vi "rotatePoints.vi"(7 "robotPos":cluster{"xPos":dbl, "yPos":dbl, "theta":dbl}, 9 "angle shift":dbl, 10 "Input":cluster{"Line":cluster{"X":dbl, "Y":dbl}[]}[](array[cluster])=[{"Line"=[{"X"=2207.719904848649, "Y"=4025.6413471932437}, {"X"=2198.7079256765874, "Y"=4062.926864756568}, {"X"=2207.699360265736, "Y"=4067.8159613100943}, {"X"=2234.0955267399086, "Y"=4039.9831033175988}, {"X"=2252.228831694671, "Y"=4026.9405312945887}, {"X"=2271.549062590683, "Y"=4011.064573925477}, {"X"=2281.5806891164716, "Y"=4012.833569019945}, {"X"=2291.606547380772, "Y"=4014.532684771267}, {"X"=2306.491333736606, "Y"=4006.2964587232555}, {"X"=2318.6274797470815, "Y"=4003.328717244889}, {"X"=2330.269715175642, "Y"=4001.167493766924}, {"X"=2341.008251095636, "Y"=4000.7261955414297}, {"X"=2355.4973825011707, "Y"=3992.0389276299557}, {"X"=2366.5383203403635, "Y"=3990.5072097629672}, {"X"=2377.53610248222, "Y"=3988.892615102757}, {"X"=2388.8934994574606, "Y"=3986.2805794624155}, {"X"=2397.411061091578, "Y"=3990.0041621179494}, {"X"=2407.911866591801, "Y"=3989.075823084253}, {"X"=2418.3785187827534, "Y"=3988.071126631001}, {"X"=2427.2873049759087, "Y"=3990.6890985976133}, {"X"=2437.3316429744427, "Y"=3990.4691007002493}, {"X"=2446.612827733287, "Y"=3992.036866455286}, {"X"=2458.074290966777, "Y"=3987.9540791715117}, {"X"=2466.9588047209436, "Y"=3990.3194180243167}, {"X"=2475.8519286932046, "Y"=3992.628019014901}, {"X"=2486.4858053530056, "Y"=3990.1896172450897}, {"X"=2497.4106848755673, "Y"=3986.733204449491}, {"X"=2506.263944361786, "Y"=3988.8486985135632}, {"X"=2516.111756914983, "Y"=3988.0749865205753}, {"X"=2525.2846850863148, "Y"=3989.1253974304846}, {"X"=2533.8171346698073, "Y"=3992.0120459509435}, {"X"=2542.367135774692, "Y"=3994.846286004641}, {"X"=2550.9343664982594, "Y"=3997.6280108840406}, {"X"=2559.8185598039045, "Y"=3999.4031941177254}, {"X"=2571.9437832226267, "Y"=3990.6088146125935}, {"X"=2582.2144175424637, "Y"=3987.463948032747}, {"X"=2590.735600977976, "Y"=3990.0013135580634}, {"X"=2599.5487477190327, "Y"=3991.5253481509435}, {"X"=2609.718442836895, "Y"=3988.1802138549383}, {"X"=2620.6261722825793, "Y"=3981.8699283373353}, {"X"=2630.4064035936003, "Y"=3979.3420799407895}, {"X"=2639.129732346304, "Y"=3980.6164021637396}, {"X"=2647.6078286155175, "Y"=3982.8046707857657}, {"X"=2656.099192250811, "Y"=3984.9408775935008}, {"X"=2664.6035035571426, "Y"=3987.0249421599656}, {"X"=2673.807645346353, "Y"=3986.136554516008}, {"X"=2686.7807721936474, "Y"=3968.6159853415393}]}, {"Line"=[{"X"=3111.693546822526, "Y"=3588.7110556670254}, {"X"=3123.438852104627, "Y"=3635.669759040541}, {"X"=3147.3373670544443, "Y"=3774.796876174543}, {"X"=3159.6335330851234, "Y"=3812.53706546017}, {"X"=3170.3490866292254, "Y"=3835.3097541445177}, {"X"=3179.3524271873403, "Y"=3844.1389419441903}, {"X"=3195.610637480107, "Y"=3900.369746843038}, {"X"=3206.0629644143296, "Y"=3914.952111180015}, {"X"=3215.736251259236, "Y"=3923.5327233931966}, {"X"=3223.853234205395, "Y"=3922.1840755113426}, {"X"=3233.691556461108, "Y"=3930.6349072674984}, {"X"=3245.0740830877103, "Y"=3946.885182114169}, {"X"=3253.3338017504625, "Y"=3945.356081076923}, {"X"=3263.30367270885, "Y"=3952.6105041504115}, {"X"=3271.5981781203227, "Y"=3950.96944067648}, {"X"=3279.8824580138976, "Y"=3949.2775139666783}, {"X"=3287.319752884467, "Y"=3943.6232208481697}, {"X"=3295.558661266366, "Y"=3941.8349666596237}, {"X"=3303.7864420317183, "Y"=3939.9961931429916}, {"X"=3311.3215566201256, "Y"=3935.1853385892246}, {"X"=3319.508239302628, "Y"=3933.249970942334}, {"X"=3334.3751764114004, "Y"=3958.45288523373}]}, {"Line"=[{"X"=3344.908865242611, "Y"=3965.101415528185}, {"X"=3352.2748452131286, "Y"=3959.0873531271145}, {"X"=3360.607416965633, "Y"=3956.9002508767453}, {"X"=3369.977484451716, "Y"=3958.521498173209}, {"X"=3378.3062509363144, "Y"=3956.2257852225457}, {"X"=3389.641249204419, "Y"=3964.456190912123}, {"X"=3400.249927965521, "Y"=3969.718582469989}, {"X"=3408.646828597577, "Y"=3967.236910515929}, {"X"=3417.0283439075047, "Y"=3964.703762864954}, {"X"=3425.39415833599, "Y"=3962.11923488864}, {"X"=3433.7439569148473, "Y"=3959.483423893006}, {"X"=3442.07742527888, "Y"=3956.7964291148455}, {"X"=3453.8661044404716, "Y"=3964.496082530115}, {"X"=3462.5513905712496, "Y"=3962.632456343457}, {"X"=3471.2308824116985, "Y"=3960.7135831840187}, {"X"=3479.5711932104623, "Y"=3957.796549797757}, {"X"=3489.5875228985537, "Y"=3959.5326614031965}, {"X"=3499.987731033616, "Y"=3962.1355544936987}, {"X"=3509.7375659322042, "Y"=3962.7885433468805}, {"X"=3522.362789825989, "Y"=3970.848684503585}, {"X"=3531.8497335130646, "Y"=3970.4144850964185}, {"X"=3540.6159427308094, "Y"=3968.055336039182}, {"X"=3549.37321102068, "Y"=3965.6401704009836}, {"X"=3558.500081793643, "Y"=3964.0944463769706}, {"X"=3569.16692785225, "Y"=3966.180444977614}, {"X"=3577.538939065994, "Y"=3962.6623844014066}, {"X"=3585.8892062651075, "Y"=3959.093020356606}, {"X"=3593.8159168133284, "Y"=3954.5566274390844}, {"X"=3602.1161416132213, "Y"=3950.8875423249738}, {"X"=3609.568283021091, "Y"=3945.3458694085766}, {"X"=3618.6482715704797, "Y"=3943.396931693257}, {"X"=3626.8795543024958, "Y"=3939.5756881929083}]}, {"Line"=[{"X"=3800.09423982062, "Y"=3947.3448732250645}, {"X"=3809.378042970595, "Y"=3944.123574511321}, {"X"=3819.694604811834, "Y"=3942.5459972911062}, {"X"=3832.6538504761256, "Y"=3945.14369689163}, {"X"=3843.5495084753843, "Y"=3944.244481763246}, {"X"=3859.2959007671043, "Y"=3950.8558601586074}, {"X"=3868.110312080752, "Y"=3946.3983385532897}, {"X"=3881.8256977872484, "Y"=3949.417444203991}, {"X"=3890.088967448885, "Y"=3943.9812610396684}, {"X"=3903.3341528929327, "Y"=3945.9674617973524}, {"X"=3914.3876190160663, "Y"=3944.533853121642}, {"X"=3929.996733704319, "Y"=3949.602561978636}, {"X"=3938.2602324211293, "Y"=3943.870803409706}, {"X"=3956.3055525432223, "Y"=3951.9673406465863}, {"X"=3970.4078429817587, "Y"=3954.2025765296307}, {"X"=3979.8737146602944, "Y"=3949.841288195704}, {"X"=3998.208687435405, "Y"=3957.499324614376}, {"X"=4008.3113782978594, "Y"=3953.754839103104}, {"X"=4017.8033817005166, "Y"=3949.1390870473633}, {"X"=4027.276658663517, "Y"=3944.457759308607}, {"X"=4044.6867826496114, "Y"=3949.9920467014626}, {"X"=4054.1841976192836, "Y"=3945.1307287731506}, {"X"=4072.364489063383, "Y"=3951.169642419422}, {"X"=4082.5142882560313, "Y"=3946.9026749255263}, {"X"=4105.907771200753, "Y"=3958.849513963111}, {"X"=4114.860669673112, "Y"=3952.809922796259}, {"X"=4127.6252414941555, "Y"=3951.3183617287414}, {"X"=4137.831733452446, "Y"=3946.665491630569}, {"X"=4155.174277321527, "Y"=3950.2967781249745}, {"X"=4169.984998772591, "Y"=3950.7420562961306}, {"X"=4185.503775549924, "Y"=3951.807973847201}, {"X"=4205.727035469534, "Y"=3957.9684517461556}, {"X"=4217.379287768711, "Y"=3954.26314640536}, {"X"=4225.665973398596, "Y"=3946.7679539003266}, {"X"=4237.972103227306, "Y"=3943.6346496093947}, {"X"=4272.112912884239, "Y"=3963.801208707917}, {"X"=4281.830236954413, "Y"=3957.4241207630703}, {"X"=4299.118370011982, "Y"=3958.9302633679963}, {"X"=4309.518481723098, "Y"=3953.0891862791714}, {"X"=4319.8957456070275, "Y"=3947.171563212521}, {"X"=4354.192697994926, "Y"=3965.3172293270245}, {"X"=4369.630150249946, "Y"=3964.0389479506475}, {"X"=4388.666973836772, "Y"=3966.128850356006}, {"X"=4404.194818830778, "Y"=3964.551541997882}, {"X"=4414.705377278174, "Y"=3957.9873694185153}, {"X"=4444.055220504324, "Y"=3969.2350127477052}, {"X"=4461.187873541066, "Y"=3968.5517886497883}, {"X"=4486.44067286851, "Y"=3975.179670458451}, {"X"=4494.850634872708, "Y"=3966.033154583249}, {"X"=4506.915932191928, "Y"=3960.185418722805}, {"X"=4515.233505756106, "Y"=3950.9135512807848}, {"X"=4497.977382829493, "Y"=3919.1208286322008}, {"X"=4462.280379962087, "Y"=3871.8412205845257}, {"X"=4470.0567239687225, "Y"=3862.8448947968027}, {"X"=4477.77772117058, "Y"=3853.8010236125533}, {"X"=4655.602195404125, "Y"=3987.2928207747054}, {"X"=4908.623903346539, "Y"=3991.4736057770633}, {"X"=4938.228890195194, "Y"=3994.923929543366}, {"X"=4946.751495910105, "Y"=3983.004921600703}, {"X"=4955.200807531504, "Y"=3971.0338443044193}, {"X"=4963.576506947583, "Y"=3959.011148358809}, {"X"=4995.824874331277, "Y"=3963.2945650154047}, {"X"=5014.931792178932, "Y"=3958.2893185424805}, {"X"=5031.554210080715, "Y"=3951.43904468656}, {"X"=5071.575746123892, "Y"=3959.800694245756}, {"X"=5100.024448915692, "Y"=3960.1107726785867}, {"X"=5142.879378726153, "Y"=3969.2760745117175}, {"X"=5159.700219994649, "Y"=3961.4345227571785}, {"X"=5176.505191252621, "Y"=3953.437901216893}, {"X"=5192.440595229726, "Y"=3944.763264068708}, {"X"=5229.741662486221, "Y"=3948.884027102843}, {"X"=5250.857959727695, "Y"=3942.862407371089}, {"X"=5284.0505064876525, "Y"=3943.731105472185}, {"X"=5306.0925039725935, "Y"=3937.7194635353917}, {"X"=5335.09070779764, "Y"=3935.459241743123}, {"X"=5366.760493308205, "Y"=3934.3664291773466}]}, {"Line"=[{"X"=5122.846755597733, "Y"=3354.672546372385}, {"X"=5117.050421618455, "Y"=3338.0118646235433}, {"X"=5109.237405226532, "Y"=3320.804112358722}, {"X"=5109.827521962431, "Y"=3306.578252969808}, {"X"=5112.222952171878, "Y"=3292.995815512847}, {"X"=5111.675019169485, "Y"=3278.4928985741553}, {"X"=5106.2592042344495, "Y"=3262.5225766550634}, {"X"=5097.860033040992, "Y"=3245.761784073082}, {"X"=5096.037668905234, "Y"=3231.147439613214}, {"X"=5099.870859474535, "Y"=3218.2745130843414}, {"X"=5102.663992924216, "Y"=3205.1017541372626}, {"X"=5104.411891461092, "Y"=3191.647353646704}, {"X"=5109.931195535304, "Y"=3179.2532693968715}, {"X"=5126.555607537422, "Y"=3155.846424879344}, {"X"=5129.926185274781, "Y"=3142.7876613196163}, {"X"=5133.216572495105, "Y"=3129.7084621112244}, {"X"=5119.902872355211, "Y"=3112.6137061961263}, {"X"=5117.167841342919, "Y"=3098.22217090708}, {"X"=5120.185020026956, "Y"=3085.2220943581315}, {"X"=5113.360892759677, "Y"=3070.0326977498703}, {"X"=5108.385479953285, "Y"=3055.367618438288}, {"X"=5102.33122299647, "Y"=3040.5762463117644}, {"X"=5104.014993194493, "Y"=3027.4691900158136}, {"X"=5056.557992678663, "Y"=3004.703870440484}, {"X"=5056.05544926616, "Y"=2991.5162698316994}, {"X"=5058.419043273326, "Y"=2978.8931805796}, {"X"=5063.6588491517905, "Y"=2966.7807987306705}, {"X"=5104.309910817449, "Y"=2960.7004286599304}, {"X"=5112.403373993726, "Y"=2948.7592085378146}, {"X"=5114.503554871097, "Y"=2935.7911798089635}, {"X"=5116.524125884749, "Y"=2922.8105087319823}, {"X"=5118.465010961325, "Y"=2909.8176840218007}, {"X"=5110.422698741624, "Y"=2895.426865122523}, {"X"=5108.230972511042, "Y"=2881.9417786443655}, {"X"=5109.921247890312, "Y"=2869.000609108957}, {"X"=5109.546630275107, "Y"=2855.8085508636073}, {"X"=5111.07653041632, "Y"=2842.8598005545487}, {"X"=5112.526949719346, "Y"=2829.901906711264}, {"X"=5106.934405419057, "Y"=2816.220746602738}, {"X"=5107.226065414028, "Y"=2803.192788355571}, {"X"=5104.449351735155, "Y"=2789.8997787820836}, {"X"=5105.574939208336, "Y"=2776.983545500179}, {"X"=5109.612196543008, "Y"=2764.293579293243}, {"X"=5110.580570140726, "Y"=2751.3461494206053}, {"X"=5108.475904803169, "Y"=2738.1968120632923}, {"X"=5110.282414482703, "Y"=2725.3161247607513}, {"X"=5110.013027915529, "Y"=2712.312163307198}, {"X"=5098.675717289241, "Y"=2698.7989557661767}, {"X"=5107.235736987412, "Y"=2686.2470217637797}, {"X"=5107.725270647045, "Y"=2673.3156427772374}, {"X"=5102.137909244258, "Y"=2660.2097211269224}, {"X"=5102.467776995775, "Y"=2647.3101119682}, {"X"=5102.718488023808, "Y"=2634.4087216105017}, {"X"=5101.890085179819, "Y"=2621.495809423548}, {"X"=5097.982446966247, "Y"=2608.5820872470404}, {"X"=5097.995611736973, "Y"=2595.7089474011377}, {"X"=5096.92982162479, "Y"=2582.844150250544}, {"X"=5095.7851836870705, "Y"=2569.9922703666066}, {"X"=5092.56223462632, "Y"=2557.19469407068}, {"X"=5092.26019431406, "Y"=2544.355779375623}, {"X"=5091.8793815880335, "Y"=2531.5189596540226}, {"X"=5094.417545822585, "Y"=2518.5681650059437}, {"X"=5093.878462657877, "Y"=2505.718593468892}, {"X"=5093.260546152515, "Y"=2492.872571573508}, {"X"=5090.567098368826, "Y"=2480.1450575998315}, {"X"=5088.79433732729, "Y"=2467.383197333639}, {"X"=5086.943711924192, "Y"=2454.6385771255846}, {"X"=5086.0125048753935, "Y"=2441.8360676276457}, {"X"=5085.002760634805, "Y"=2429.0395129123663}, {"X"=5083.914517218727, "Y"=2416.249394762798}, {"X"=5084.738970298335, "Y"=2403.278303892433}, {"X"=5084.487646211095, "Y"=2390.3902368845256}, {"X"=5088.134012641568, "Y"=2377.0732289530392}, {"X"=5081.758453891878, "Y"=2364.826150157596}, {"X"=5085.241125584982, "Y"=2351.4653984470597}, {"X"=5083.676891863632, "Y"=2338.675278028435}, {"X"=5090.957212637366, "Y"=2324.7202606079113}, {"X"=5091.210016839676, "Y"=2311.622356155337}, {"X"=5096.3295775957, "Y"=2297.7975809206155}, {"X"=5097.402458596262, "Y"=2284.4941733115534}, {"X"=5095.42706822901, "Y"=2271.6306930707788}, {"X"=5097.320683975051, "Y"=2258.136067169369}, {"X"=5095.183564848325, "Y"=2245.273584872137}, {"X"=5093.9524891567, "Y"=2232.251481098212}, {"X"=5091.656608600966, "Y"=2219.4101529258787}, {"X"=5091.247436473114, "Y"=2206.2130532322985}, {"X"=5089.773413161267, "Y"=2193.1977364316826}, {"X"=5087.237982003067, "Y"=2180.382785763304}, {"X"=5088.540593099364, "Y"=2166.771202508242}, {"X"=5085.843034984822, "Y"=2153.964313753589}, {"X"=5087.949897174873, "Y"=2140.0986770105606}, {"X"=5091.915454360784, "Y"=2125.748240059654}, {"X"=5088.9661205498805, "Y"=2112.9214157912693}, {"X"=5072.323623689361, "Y"=2103.3755959490154}, {"X"=5082.831621748643, "Y"=2087.3232641869527}, {"X"=5084.494348995453, "Y"=2073.328082193457}, {"X"=5062.831303072565, "Y"=2065.315031945031}, {"X"=5079.807222141564, "Y"=2047.274101631024}, {"X"=5083.130621133493, "Y"=2032.6836726340523}, {"X"=5079.610419243946, "Y"=2019.9125030031942}, {"X"=5071.2041122091, "Y"=2008.5361164296557}, {"X"=5080.973992147818, "Y"=1991.9118123130706}, {"X"=5086.784857115412, "Y"=1976.2909651818343}]}, {"Line"=[{"X"=5076.554590880745, "Y"=1923.4077807925203}, {"X"=5072.364008515835, "Y"=1910.6790180125245}, {"X"=5064.30768229933, "Y"=1899.2619656391078}, {"X"=5062.80399450744, "Y"=1885.6270720105986}, {"X"=5058.381852922572, "Y"=1872.9833925149728}, {"X"=5059.527332741589, "Y"=1858.3341954152704}, {"X"=5057.75405613383, "Y"=1844.6773904716156}, {"X"=5053.080747090284, "Y"=1832.065467681518}, {"X"=5066.08482715571, "Y"=1812.7170222868021}, {"X"=5064.012020410524, "Y"=1798.9691768721605}, {"X"=5066.498271025875, "Y"=1783.3795888865689}, {"X"=5061.448681135181, "Y"=1770.7151665163383}, {"X"=5056.321478866777, "Y"=1758.0819662513745}, {"X"=5051.116857256931, "Y"=1745.4804637245277}, {"X"=5049.517883565899, "Y"=1731.3502173237152}, {"X"=5044.1493671039225, "Y"=1718.7909640904531}, {"X"=5059.768664712983, "Y"=1697.0304280505916}, {"X"=5060.583026021055, "Y"=1681.5591511295288}, {"X"=5057.641380496936, "Y"=1667.6948196718724}, {"X"=5085.489760086355, "Y"=1639.6102558987013}, {"X"=5079.557660642947, "Y"=1626.8320103593444}, {"X"=5078.062831634885, "Y"=1611.9433883741262}, {"X"=5077.363878206984, "Y"=1596.6016157473446}, {"X"=5074.75913760187, "Y"=1582.1122257647717}, {"X"=5079.215110997742, "Y"=1564.0494595789582}, {"X"=5072.8194973426125, "Y"=1551.3111369732596}]}, {"Line"=[{"X"=4089.4488167978225, "Y"=-45.45313237218852}, {"X"=4073.196112966746, "Y"=-52.088064735608896}, {"X"=4056.9030039085883, "Y"=-58.62314748235849}, {"X"=4039.842685990593, "Y"=-63.19510896063866}, {"X"=4021.6921231205024, "Y"=-64.85669512518461}, {"X"=4003.208136479673, "Y"=-65.46007940486334}, {"X"=3980.25078046987, "Y"=-53.742528465828855}, {"X"=3962.9270539265403, "Y"=-56.88680391475327}, {"X"=3944.931759128495, "Y"=-58.034042406215576}, {"X"=3924.325296995053, "Y"=-51.50650486379254}, {"X"=3906.421680996634, "Y"=-52.3967908703321}, {"X"=3888.8595640730305, "Y"=-54.1156107743127}, {"X"=3870.687050259731, "Y"=-53.81858093389792}, {"X"=3854.387135129674, "Y"=-59.11105885499046}, {"X"=3833.5542200850396, "Y"=-49.9945966319292}, {"X"=3817.2784674965933, "Y"=-55.05930377579716}, {"X"=3800.1069643337914, "Y"=-57.15145327182381}, {"X"=3778.4214518320896, "Y"=-43.7844169537766}]}, {"Line"=[{"X"=3753.3350906169576, "Y"=-17.759011300532165}, {"X"=3737.258641964145, "Y"=-22.33210994511228}, {"X"=3721.1544359401632, "Y"=-26.806479267901068}, {"X"=3705.799535994574, "Y"=-34.079728290289495}, {"X"=3695.4402495078234, "Y"=-60.61324873881222}, {"X"=3679.1019420513853, "Y"=-64.83030459765632}, {"X"=3662.7380667906586, "Y"=-68.9470311017003}, {"X"=3646.3492398162985, "Y"=-72.96327325851826}, {"X"=3629.9360781583773, "Y"=-76.87887985886346}, {"X"=3612.160656054581, "Y"=-74.8449172202163}, {"X"=3595.3023820924454, "Y"=-76.59841475613575}, {"X"=3577.8123188064874, "Y"=-75.31342542055609}, {"X"=3561.3860270741616, "Y"=-78.80845313842656}, {"X"=3544.938599475213, "Y"=-82.20262523210477}, {"X"=3527.312151800077, "Y"=-79.60872042243727}, {"X"=3510.6733954326514, "Y"=-81.81145556455704}, {"X"=3494.208496408174, "Y"=-84.89440426955571}, {"X"=3476.6750456786003, "Y"=-81.96884784803296}, {"X"=3458.6893038930734, "Y"=-75.97255637909848}, {"X"=3442.261210266309, "Y"=-78.73664661044631}, {"X"=3420.3271190509204, "Y"=-46.83303458876162}, {"X"=3404.0785443258815, "Y"=-49.3622874222915}, {"X"=3387.814756272034, "Y"=-51.79179326312533}, {"X"=3372.2295320760086, "Y"=-59.0731797847302}, {"X"=3357.6299571144796, "Y"=-74.1923666360085}, {"X"=3341.5940974157465, "Y"=-79.31231337646068}, {"X"=3325.7496181820807, "Y"=-86.321497187972}, {"X"=3309.2605272002866, "Y"=-88.26969002661644}, {"X"=3292.867981867008, "Y"=-91.11080136012743}, {"X"=3278.800216700698, "Y"=-116.73175694024758}, {"X"=3262.50934159305, "Y"=-122.37283368321596}, {"X"=3245.8002342494074, "Y"=-123.93231282330817}, {"X"=3231.4271349820133, "Y"=-153.29084573243335}, {"X"=3215.5382684867877, "Y"=-167.61978147608215}, {"X"=3198.5524153079396, "Y"=-168.8901997687417}, {"X"=3180.708846062885, "Y"=-157.0842049082612}, {"X"=3163.788293620604, "Y"=-158.1411122117829}, {"X"=3146.648962879583, "Y"=-155.0998315281322}, {"X"=3129.7412274911385, "Y"=-155.94778867254536}, {"X"=3112.828607418809, "Y"=-156.6919859403829}, {"X"=3097.6151374672754, "Y"=-206.30277855709028}, {"X"=3078.991260384774, "Y"=-157.86899267946092}, {"X"=3061.8653389978836, "Y"=-149.30403553893575}]}, {"Line"=[{"X"=2038.9622454495147, "Y"=-18.191634378309118}, {"X"=2022.9154148557272, "Y"=-12.24553085529169}, {"X"=2006.90537094432, "Y"=-6.20107776448458}, {"X"=1990.5709139445926, "Y"=-0.9907574278972788}, {"X"=1970.9553775348306, "Y"=-4.048226315233933}, {"X"=1953.8769629816818, "Y"=-0.46834078393840173}, {"X"=1933.393670115941, "Y"=-5.105743928882475}, {"X"=1917.0445480865305, "Y"=0.5647749615122848}, {"X"=1896.0421225556117, "Y"=-4.710733426742991}, {"X"=1880.080699645954, "Y"=2.112057710243789}, {"X"=1863.75994281155, "Y"=8.116798071258017}, {"X"=1843.8067328049035, "Y"=6.003637455763965}, {"X"=1826.2612072363017, "Y"=9.503281924175553}, {"X"=1803.277413818025, "Y"=1.312629091000872}, {"X"=1786.506988527354, "Y"=6.893039015349586}, {"X"=1765.0365862511896, "Y"=2.6472386866885245}, {"X"=1749.1227771518695, "Y"=10.273726171094495}, {"X"=1731.9347027160445, "Y"=15.304388941677644}, {"X"=1713.4234571180775, "Y"=17.763411438448202}, {"X"=1693.0889976485528, "Y"=16.783278171818893}, {"X"=1677.2632800499323, "Y"=24.8509616537267}, {"X"=1651.3155914045235, "Y"=13.508289978205084}, {"X"=1631.2604984090294, "Y"=13.877772265103886}, {"X"=1606.9005249663614, "Y"=6.467688140168775}, {"X"=1585.748577668781, "Y"=5.406021275366584}, {"X"=1564.0473760449063, "Y"=3.631562786883478}, {"X"=1543.2500413395983, "Y"=3.770318723145465}, {"X"=1526.8526216432042, "Y"=11.888564678773491}, {"X"=1504.5000000000007, "Y"=9.71801728074388}]}]) -> (2 "Output":cluster{"Line":cluster{"X":dbl, "Y":dbl}[]}[](array[cluster])=[{"Line"=[{"X"=2207.719904848649, "Y"=4025.6413471932437}, {"X"=2198.7079256765874, "Y"=4062.926864756568}, {"X"=2207.699360265736, "Y"=4067.8159613100943}, {"X"=2234.0955267399086, "Y"=4039.9831033175988}, {"X"=2252.228831694671, "Y"=4026.9405312945887}, {"X"=2271.549062590683, "Y"=4011.064573925477}, {"X"=2281.5806891164716, "Y"=4012.833569019945}, {"X"=2291.606547380772, "Y"=4014.532684771267}, {"X"=2306.491333736606, "Y"=4006.2964587232555}, {"X"=2318.6274797470815, "Y"=4003.328717244889}, {"X"=2330.269715175642, "Y"=4001.167493766924}, {"X"=2341.008251095636, "Y"=4000.7261955414297}, {"X"=2355.4973825011707, "Y"=3992.0389276299557}, {"X"=2366.5383203403635, "Y"=3990.5072097629672}, {"X"=2377.53610248222, "Y"=3988.892615102757}, {"X"=2388.8934994574606, "Y"=3986.2805794624155}, {"X"=2397.411061091578, "Y"=3990.0041621179494}, {"X"=2407.911866591801, "Y"=3989.075823084253}, {"X"=2418.3785187827534, "Y"=3988.071126631001}, {"X"=2427.2873049759087, "Y"=3990.6890985976133}, {"X"=2437.3316429744427, "Y"=3990.4691007002493}, {"X"=2446.612827733287, "Y"=3992.036866455286}, {"X"=2458.074290966777, "Y"=3987.9540791715117}, {"X"=2466.9588047209436, "Y"=3990.3194180243167}, {"X"=2475.8519286932046, "Y"=3992.628019014901}, {"X"=2486.4858053530056, "Y"=3990.1896172450897}, {"X"=2497.4106848755673, "Y"=3986.733204449491}, {"X"=2506.263944361786, "Y"=3988.8486985135632}, {"X"=2516.111756914983, "Y"=3988.0749865205753}, {"X"=2525.2846850863148, "Y"=3989.1253974304846}, {"X"=2533.8171346698073, "Y"=3992.0120459509435}, {"X"=2542.367135774692, "Y"=3994.846286004641}, {"X"=2550.9343664982594, "Y"=3997.6280108840406}, {"X"=2559.8185598039045, "Y"=3999.4031941177254}, {"X"=2571.9437832226267, "Y"=3990.6088146125935}, {"X"=2582.2144175424637, "Y"=3987.463948032747}, {"X"=2590.735600977976, "Y"=3990.0013135580634}, {"X"=2599.5487477190327, "Y"=3991.5253481509435}, {"X"=2609.718442836895, "Y"=3988.1802138549383}, {"X"=2620.6261722825793, "Y"=3981.8699283373353}, {"X"=2630.4064035936003, "Y"=3979.3420799407895}, {"X"=2639.129732346304, "Y"=3980.6164021637396}, {"X"=2647.6078286155175, "Y"=3982.8046707857657}, {"X"=2656.099192250811, "Y"=3984.9408775935008}, {"X"=2664.6035035571426, "Y"=3987.0249421599656}, {"X"=2673.807645346353, "Y"=3986.136554516008}, {"X"=2686.7807721936474, "Y"=3968.6159853415393}]}, {"Line"=[{"X"=3111.693546822526, "Y"=3588.7110556670254}, {"X"=3123.438852104627, "Y"=3635.669759040541}, {"X"=3147.3373670544443, "Y"=3774.796876174543}, {"X"=3159.6335330851234, "Y"=3812.53706546017}, {"X"=3170.3490866292254, "Y"=3835.3097541445177}, {"X"=3179.3524271873403, "Y"=3844.1389419441903}, {"X"=3195.610637480107, "Y"=3900.369746843038}, {"X"=3206.0629644143296, "Y"=3914.952111180015}, {"X"=3215.736251259236, "Y"=3923.5327233931966}, {"X"=3223.853234205395, "Y"=3922.1840755113426}, {"X"=3233.691556461108, "Y"=3930.6349072674984}, {"X"=3245.0740830877103, "Y"=3946.885182114169}, {"X"=3253.3338017504625, "Y"=3945.356081076923}, {"X"=3263.30367270885, "Y"=3952.6105041504115}, {"X"=3271.5981781203227, "Y"=3950.96944067648}, {"X"=3279.8824580138976, "Y"=3949.2775139666783}, {"X"=3287.319752884467, "Y"=3943.6232208481697}, {"X"=3295.558661266366, "Y"=3941.8349666596237}, {"X"=3303.7864420317183, "Y"=3939.9961931429916}, {"X"=3311.3215566201256, "Y"=3935.1853385892246}, {"X"=3319.508239302628, "Y"=3933.249970942334}, {"X"=3334.3751764114004, "Y"=3958.45288523373}]}, {"Line"=[{"X"=3344.908865242611, "Y"=3965.101415528185}, {"X"=3352.2748452131286, "Y"=3959.0873531271145}, {"X"=3360.607416965633, "Y"=3956.9002508767453}, {"X"=3369.977484451716, "Y"=3958.521498173209}, {"X"=3378.3062509363144, "Y"=3956.2257852225457}, {"X"=3389.641249204419, "Y"=3964.456190912123}, {"X"=3400.249927965521, "Y"=3969.718582469989}, {"X"=3408.646828597577, "Y"=3967.236910515929}, {"X"=3417.0283439075047, "Y"=3964.703762864954}, {"X"=3425.39415833599, "Y"=3962.11923488864}, {"X"=3433.7439569148473, "Y"=3959.483423893006}, {"X"=3442.07742527888, "Y"=3956.7964291148455}, {"X"=3453.8661044404716, "Y"=3964.496082530115}, {"X"=3462.5513905712496, "Y"=3962.632456343457}, {"X"=3471.2308824116985, "Y"=3960.7135831840187}, {"X"=3479.5711932104623, "Y"=3957.796549797757}, {"X"=3489.5875228985537, "Y"=3959.5326614031965}, {"X"=3499.987731033616, "Y"=3962.1355544936987}, {"X"=3509.7375659322042, "Y"=3962.7885433468805}, {"X"=3522.362789825989, "Y"=3970.848684503585}, {"X"=3531.8497335130646, "Y"=3970.4144850964185}, {"X"=3540.6159427308094, "Y"=3968.055336039182}, {"X"=3549.37321102068, "Y"=3965.6401704009836}, {"X"=3558.500081793643, "Y"=3964.0944463769706}, {"X"=3569.16692785225, "Y"=3966.180444977614}, {"X"=3577.538939065994, "Y"=3962.6623844014066}, {"X"=3585.8892062651075, "Y"=3959.093020356606}, {"X"=3593.8159168133284, "Y"=3954.5566274390844}, {"X"=3602.1161416132213, "Y"=3950.8875423249738}, {"X"=3609.568283021091, "Y"=3945.3458694085766}, {"X"=3618.6482715704797, "Y"=3943.396931693257}, {"X"=3626.8795543024958, "Y"=3939.5756881929083}]}, {"Line"=[{"X"=3800.09423982062, "Y"=3947.3448732250645}, {"X"=3809.378042970595, "Y"=3944.123574511321}, {"X"=3819.694604811834, "Y"=3942.5459972911062}, {"X"=3832.6538504761256, "Y"=3945.14369689163}, {"X"=3843.5495084753843, "Y"=3944.244481763246}, {"X"=3859.2959007671043, "Y"=3950.8558601586074}, {"X"=3868.110312080752, "Y"=3946.3983385532897}, {"X"=3881.8256977872484, "Y"=3949.417444203991}, {"X"=3890.088967448885, "Y"=3943.9812610396684}, {"X"=3903.3341528929327, "Y"=3945.9674617973524}, {"X"=3914.3876190160663, "Y"=3944.533853121642}, {"X"=3929.996733704319, "Y"=3949.602561978636}, {"X"=3938.2602324211293, "Y"=3943.870803409706}, {"X"=3956.3055525432223, "Y"=3951.9673406465863}, {"X"=3970.4078429817587, "Y"=3954.2025765296307}, {"X"=3979.8737146602944, "Y"=3949.841288195704}, {"X"=3998.208687435405, "Y"=3957.499324614376}, {"X"=4008.3113782978594, "Y"=3953.754839103104}, {"X"=4017.8033817005166, "Y"=3949.1390870473633}, {"X"=4027.276658663517, "Y"=3944.457759308607}, {"X"=4044.6867826496114, "Y"=3949.9920467014626}, {"X"=4054.1841976192836, "Y"=3945.1307287731506}, {"X"=4072.364489063383, "Y"=3951.169642419422}, {"X"=4082.5142882560313, "Y"=3946.9026749255263}, {"X"=4105.907771200753, "Y"=3958.849513963111}, {"X"=4114.860669673112, "Y"=3952.809922796259}, {"X"=4127.6252414941555, "Y"=3951.3183617287414}, {"X"=4137.831733452446, "Y"=3946.665491630569}, {"X"=4155.174277321527, "Y"=3950.2967781249745}, {"X"=4169.984998772591, "Y"=3950.7420562961306}, {"X"=4185.503775549924, "Y"=3951.807973847201}, {"X"=4205.727035469534, "Y"=3957.9684517461556}, {"X"=4217.379287768711, "Y"=3954.26314640536}, {"X"=4225.665973398596, "Y"=3946.7679539003266}, {"X"=4237.972103227306, "Y"=3943.6346496093947}, {"X"=4272.112912884239, "Y"=3963.801208707917}, {"X"=4281.830236954413, "Y"=3957.4241207630703}, {"X"=4299.118370011982, "Y"=3958.9302633679963}, {"X"=4309.518481723098, "Y"=3953.0891862791714}, {"X"=4319.8957456070275, "Y"=3947.171563212521}, {"X"=4354.192697994926, "Y"=3965.3172293270245}, {"X"=4369.630150249946, "Y"=3964.0389479506475}, {"X"=4388.666973836772, "Y"=3966.128850356006}, {"X"=4404.194818830778, "Y"=3964.551541997882}, {"X"=4414.705377278174, "Y"=3957.9873694185153}, {"X"=4444.055220504324, "Y"=3969.2350127477052}, {"X"=4461.187873541066, "Y"=3968.5517886497883}, {"X"=4486.44067286851, "Y"=3975.179670458451}, {"X"=4494.850634872708, "Y"=3966.033154583249}, {"X"=4506.915932191928, "Y"=3960.185418722805}, {"X"=4515.233505756106, "Y"=3950.9135512807848}, {"X"=4497.977382829493, "Y"=3919.1208286322008}, {"X"=4462.280379962087, "Y"=3871.8412205845257}, {"X"=4470.0567239687225, "Y"=3862.8448947968027}, {"X"=4477.77772117058, "Y"=3853.8010236125533}, {"X"=4655.602195404125, "Y"=3987.2928207747054}, {"X"=4908.623903346539, "Y"=3991.4736057770633}, {"X"=4938.228890195194, "Y"=3994.923929543366}, {"X"=4946.751495910105, "Y"=3983.004921600703}, {"X"=4955.200807531504, "Y"=3971.0338443044193}, {"X"=4963.576506947583, "Y"=3959.011148358809}, {"X"=4995.824874331277, "Y"=3963.2945650154047}, {"X"=5014.931792178932, "Y"=3958.2893185424805}, {"X"=5031.554210080715, "Y"=3951.43904468656}, {"X"=5071.575746123892, "Y"=3959.800694245756}, {"X"=5100.024448915692, "Y"=3960.1107726785867}, {"X"=5142.879378726153, "Y"=3969.2760745117175}, {"X"=5159.700219994649, "Y"=3961.4345227571785}, {"X"=5176.505191252621, "Y"=3953.437901216893}, {"X"=5192.440595229726, "Y"=3944.763264068708}, {"X"=5229.741662486221, "Y"=3948.884027102843}, {"X"=5250.857959727695, "Y"=3942.862407371089}, {"X"=5284.0505064876525, "Y"=3943.731105472185}, {"X"=5306.0925039725935, "Y"=3937.7194635353917}, {"X"=5335.09070779764, "Y"=3935.459241743123}, {"X"=5366.760493308205, "Y"=3934.3664291773466}]}, {"Line"=[{"X"=5122.846755597733, "Y"=3354.672546372385}, {"X"=5117.050421618455, "Y"=3338.0118646235433}, {"X"=5109.237405226532, "Y"=3320.804112358722}, {"X"=5109.827521962431, "Y"=3306.578252969808}, {"X"=5112.222952171878, "Y"=3292.995815512847}, {"X"=5111.675019169485, "Y"=3278.4928985741553}, {"X"=5106.2592042344495, "Y"=3262.5225766550634}, {"X"=5097.860033040992, "Y"=3245.761784073082}, {"X"=5096.037668905234, "Y"=3231.147439613214}, {"X"=5099.870859474535, "Y"=3218.2745130843414}, {"X"=5102.663992924216, "Y"=3205.1017541372626}, {"X"=5104.411891461092, "Y"=3191.647353646704}, {"X"=5109.931195535304, "Y"=3179.2532693968715}, {"X"=5126.555607537422, "Y"=3155.846424879344}, {"X"=5129.926185274781, "Y"=3142.7876613196163}, {"X"=5133.216572495105, "Y"=3129.7084621112244}, {"X"=5119.902872355211, "Y"=3112.6137061961263}, {"X"=5117.167841342919, "Y"=3098.22217090708}, {"X"=5120.185020026956, "Y"=3085.2220943581315}, {"X"=5113.360892759677, "Y"=3070.0326977498703}, {"X"=5108.385479953285, "Y"=3055.367618438288}, {"X"=5102.33122299647, "Y"=3040.5762463117644}, {"X"=5104.014993194493, "Y"=3027.4691900158136}, {"X"=5056.557992678663, "Y"=3004.703870440484}, {"X"=5056.05544926616, "Y"=2991.5162698316994}, {"X"=5058.419043273326, "Y"=2978.8931805796}, {"X"=5063.6588491517905, "Y"=2966.7807987306705}, {"X"=5104.309910817449, "Y"=2960.7004286599304}, {"X"=5112.403373993726, "Y"=2948.7592085378146}, {"X"=5114.503554871097, "Y"=2935.7911798089635}, {"X"=5116.524125884749, "Y"=2922.8105087319823}, {"X"=5118.465010961325, "Y"=2909.8176840218007}, {"X"=5110.422698741624, "Y"=2895.426865122523}, {"X"=5108.230972511042, "Y"=2881.9417786443655}, {"X"=5109.921247890312, "Y"=2869.000609108957}, {"X"=5109.546630275107, "Y"=2855.8085508636073}, {"X"=5111.07653041632, "Y"=2842.8598005545487}, {"X"=5112.526949719346, "Y"=2829.901906711264}, {"X"=5106.934405419057, "Y"=2816.220746602738}, {"X"=5107.226065414028, "Y"=2803.192788355571}, {"X"=5104.449351735155, "Y"=2789.8997787820836}, {"X"=5105.574939208336, "Y"=2776.983545500179}, {"X"=5109.612196543008, "Y"=2764.293579293243}, {"X"=5110.580570140726, "Y"=2751.3461494206053}, {"X"=5108.475904803169, "Y"=2738.1968120632923}, {"X"=5110.282414482703, "Y"=2725.3161247607513}, {"X"=5110.013027915529, "Y"=2712.312163307198}, {"X"=5098.675717289241, "Y"=2698.7989557661767}, {"X"=5107.235736987412, "Y"=2686.2470217637797}, {"X"=5107.725270647045, "Y"=2673.3156427772374}, {"X"=5102.137909244258, "Y"=2660.2097211269224}, {"X"=5102.467776995775, "Y"=2647.3101119682}, {"X"=5102.718488023808, "Y"=2634.4087216105017}, {"X"=5101.890085179819, "Y"=2621.495809423548}, {"X"=5097.982446966247, "Y"=2608.5820872470404}, {"X"=5097.995611736973, "Y"=2595.7089474011377}, {"X"=5096.92982162479, "Y"=2582.844150250544}, {"X"=5095.7851836870705, "Y"=2569.9922703666066}, {"X"=5092.56223462632, "Y"=2557.19469407068}, {"X"=5092.26019431406, "Y"=2544.355779375623}, {"X"=5091.8793815880335, "Y"=2531.5189596540226}, {"X"=5094.417545822585, "Y"=2518.5681650059437}, {"X"=5093.878462657877, "Y"=2505.718593468892}, {"X"=5093.260546152515, "Y"=2492.872571573508}, {"X"=5090.567098368826, "Y"=2480.1450575998315}, {"X"=5088.79433732729, "Y"=2467.383197333639}, {"X"=5086.943711924192, "Y"=2454.6385771255846}, {"X"=5086.0125048753935, "Y"=2441.8360676276457}, {"X"=5085.002760634805, "Y"=2429.0395129123663}, {"X"=5083.914517218727, "Y"=2416.249394762798}, {"X"=5084.738970298335, "Y"=2403.278303892433}, {"X"=5084.487646211095, "Y"=2390.3902368845256}, {"X"=5088.134012641568, "Y"=2377.0732289530392}, {"X"=5081.758453891878, "Y"=2364.826150157596}, {"X"=5085.241125584982, "Y"=2351.4653984470597}, {"X"=5083.676891863632, "Y"=2338.675278028435}, {"X"=5090.957212637366, "Y"=2324.7202606079113}, {"X"=5091.210016839676, "Y"=2311.622356155337}, {"X"=5096.3295775957, "Y"=2297.7975809206155}, {"X"=5097.402458596262, "Y"=2284.4941733115534}, {"X"=5095.42706822901, "Y"=2271.6306930707788}, {"X"=5097.320683975051, "Y"=2258.136067169369}, {"X"=5095.183564848325, "Y"=2245.273584872137}, {"X"=5093.9524891567, "Y"=2232.251481098212}, {"X"=5091.656608600966, "Y"=2219.4101529258787}, {"X"=5091.247436473114, "Y"=2206.2130532322985}, {"X"=5089.773413161267, "Y"=2193.1977364316826}, {"X"=5087.237982003067, "Y"=2180.382785763304}, {"X"=5088.540593099364, "Y"=2166.771202508242}, {"X"=5085.843034984822, "Y"=2153.964313753589}, {"X"=5087.949897174873, "Y"=2140.0986770105606}, {"X"=5091.915454360784, "Y"=2125.748240059654}, {"X"=5088.9661205498805, "Y"=2112.9214157912693}, {"X"=5072.323623689361, "Y"=2103.3755959490154}, {"X"=5082.831621748643, "Y"=2087.3232641869527}, {"X"=5084.494348995453, "Y"=2073.328082193457}, {"X"=5062.831303072565, "Y"=2065.315031945031}, {"X"=5079.807222141564, "Y"=2047.274101631024}, {"X"=5083.130621133493, "Y"=2032.6836726340523}, {"X"=5079.610419243946, "Y"=2019.9125030031942}, {"X"=5071.2041122091, "Y"=2008.5361164296557}, {"X"=5080.973992147818, "Y"=1991.9118123130706}, {"X"=5086.784857115412, "Y"=1976.2909651818343}]}, {"Line"=[{"X"=5076.554590880745, "Y"=1923.4077807925203}, {"X"=5072.364008515835, "Y"=1910.6790180125245}, {"X"=5064.30768229933, "Y"=1899.2619656391078}, {"X"=5062.80399450744, "Y"=1885.6270720105986}, {"X"=5058.381852922572, "Y"=1872.9833925149728}, {"X"=5059.527332741589, "Y"=1858.3341954152704}, {"X"=5057.75405613383, "Y"=1844.6773904716156}, {"X"=5053.080747090284, "Y"=1832.065467681518}, {"X"=5066.08482715571, "Y"=1812.7170222868021}, {"X"=5064.012020410524, "Y"=1798.9691768721605}, {"X"=5066.498271025875, "Y"=1783.3795888865689}, {"X"=5061.448681135181, "Y"=1770.7151665163383}, {"X"=5056.321478866777, "Y"=1758.0819662513745}, {"X"=5051.116857256931, "Y"=1745.4804637245277}, {"X"=5049.517883565899, "Y"=1731.3502173237152}, {"X"=5044.1493671039225, "Y"=1718.7909640904531}, {"X"=5059.768664712983, "Y"=1697.0304280505916}, {"X"=5060.583026021055, "Y"=1681.5591511295288}, {"X"=5057.641380496936, "Y"=1667.6948196718724}, {"X"=5085.489760086355, "Y"=1639.6102558987013}, {"X"=5079.557660642947, "Y"=1626.8320103593444}, {"X"=5078.062831634885, "Y"=1611.9433883741262}, {"X"=5077.363878206984, "Y"=1596.6016157473446}, {"X"=5074.75913760187, "Y"=1582.1122257647717}, {"X"=5079.215110997742, "Y"=1564.0494595789582}, {"X"=5072.8194973426125, "Y"=1551.3111369732596}]}, {"Line"=[{"X"=4089.4488167978225, "Y"=-45.45313237218852}, {"X"=4073.196112966746, "Y"=-52.088064735608896}, {"X"=4056.9030039085883, "Y"=-58.62314748235849}, {"X"=4039.842685990593, "Y"=-63.19510896063866}, {"X"=4021.6921231205024, "Y"=-64.85669512518461}, {"X"=4003.208136479673, "Y"=-65.46007940486334}, {"X"=3980.25078046987, "Y"=-53.742528465828855}, {"X"=3962.9270539265403, "Y"=-56.88680391475327}, {"X"=3944.931759128495, "Y"=-58.034042406215576}, {"X"=3924.325296995053, "Y"=-51.50650486379254}, {"X"=3906.421680996634, "Y"=-52.3967908703321}, {"X"=3888.8595640730305, "Y"=-54.1156107743127}, {"X"=3870.687050259731, "Y"=-53.81858093389792}, {"X"=3854.387135129674, "Y"=-59.11105885499046}, {"X"=3833.5542200850396, "Y"=-49.9945966319292}, {"X"=3817.2784674965933, "Y"=-55.05930377579716}, {"X"=3800.1069643337914, "Y"=-57.15145327182381}, {"X"=3778.4214518320896, "Y"=-43.7844169537766}]}, {"Line"=[{"X"=3753.3350906169576, "Y"=-17.759011300532165}, {"X"=3737.258641964145, "Y"=-22.33210994511228}, {"X"=3721.1544359401632, "Y"=-26.806479267901068}, {"X"=3705.799535994574, "Y"=-34.079728290289495}, {"X"=3695.4402495078234, "Y"=-60.61324873881222}, {"X"=3679.1019420513853, "Y"=-64.83030459765632}, {"X"=3662.7380667906586, "Y"=-68.9470311017003}, {"X"=3646.3492398162985, "Y"=-72.96327325851826}, {"X"=3629.9360781583773, "Y"=-76.87887985886346}, {"X"=3612.160656054581, "Y"=-74.8449172202163}, {"X"=3595.3023820924454, "Y"=-76.59841475613575}, {"X"=3577.8123188064874, "Y"=-75.31342542055609}, {"X"=3561.3860270741616, "Y"=-78.80845313842656}, {"X"=3544.938599475213, "Y"=-82.20262523210477}, {"X"=3527.312151800077, "Y"=-79.60872042243727}, {"X"=3510.6733954326514, "Y"=-81.81145556455704}, {"X"=3494.208496408174, "Y"=-84.89440426955571}, {"X"=3476.6750456786003, "Y"=-81.96884784803296}, {"X"=3458.6893038930734, "Y"=-75.97255637909848}, {"X"=3442.261210266309, "Y"=-78.73664661044631}, {"X"=3420.3271190509204, "Y"=-46.83303458876162}, {"X"=3404.0785443258815, "Y"=-49.3622874222915}, {"X"=3387.814756272034, "Y"=-51.79179326312533}, {"X"=3372.2295320760086, "Y"=-59.0731797847302}, {"X"=3357.6299571144796, "Y"=-74.1923666360085}, {"X"=3341.5940974157465, "Y"=-79.31231337646068}, {"X"=3325.7496181820807, "Y"=-86.321497187972}, {"X"=3309.2605272002866, "Y"=-88.26969002661644}, {"X"=3292.867981867008, "Y"=-91.11080136012743}, {"X"=3278.800216700698, "Y"=-116.73175694024758}, {"X"=3262.50934159305, "Y"=-122.37283368321596}, {"X"=3245.8002342494074, "Y"=-123.93231282330817}, {"X"=3231.4271349820133, "Y"=-153.29084573243335}, {"X"=3215.5382684867877, "Y"=-167.61978147608215}, {"X"=3198.5524153079396, "Y"=-168.8901997687417}, {"X"=3180.708846062885, "Y"=-157.0842049082612}, {"X"=3163.788293620604, "Y"=-158.1411122117829}, {"X"=3146.648962879583, "Y"=-155.0998315281322}, {"X"=3129.7412274911385, "Y"=-155.94778867254536}, {"X"=3112.828607418809, "Y"=-156.6919859403829}, {"X"=3097.6151374672754, "Y"=-206.30277855709028}, {"X"=3078.991260384774, "Y"=-157.86899267946092}, {"X"=3061.8653389978836, "Y"=-149.30403553893575}]}, {"Line"=[{"X"=2038.9622454495147, "Y"=-18.191634378309118}, {"X"=2022.9154148557272, "Y"=-12.24553085529169}, {"X"=2006.90537094432, "Y"=-6.20107776448458}, {"X"=1990.5709139445926, "Y"=-0.9907574278972788}, {"X"=1970.9553775348306, "Y"=-4.048226315233933}, {"X"=1953.8769629816818, "Y"=-0.46834078393840173}, {"X"=1933.393670115941, "Y"=-5.105743928882475}, {"X"=1917.0445480865305, "Y"=0.5647749615122848}, {"X"=1896.0421225556117, "Y"=-4.710733426742991}, {"X"=1880.080699645954, "Y"=2.112057710243789}, {"X"=1863.75994281155, "Y"=8.116798071258017}, {"X"=1843.8067328049035, "Y"=6.003637455763965}, {"X"=1826.2612072363017, "Y"=9.503281924175553}, {"X"=1803.277413818025, "Y"=1.312629091000872}, {"X"=1786.506988527354, "Y"=6.893039015349586}, {"X"=1765.0365862511896, "Y"=2.6472386866885245}, {"X"=1749.1227771518695, "Y"=10.273726171094495}, {"X"=1731.9347027160445, "Y"=15.304388941677644}, {"X"=1713.4234571180775, "Y"=17.763411438448202}, {"X"=1693.0889976485528, "Y"=16.783278171818893}, {"X"=1677.2632800499323, "Y"=24.8509616537267}, {"X"=1651.3155914045235, "Y"=13.508289978205084}, {"X"=1631.2604984090294, "Y"=13.877772265103886}, {"X"=1606.9005249663614, "Y"=6.467688140168775}, {"X"=1585.748577668781, "Y"=5.406021275366584}, {"X"=1564.0473760449063, "Y"=3.631562786883478}, {"X"=1543.2500413395983, "Y"=3.770318723145465}, {"X"=1526.8526216432042, "Y"=11.888564678773491}, {"X"=1504.5000000000007, "Y"=9.71801728074388}]}])   [LabVIEW 2016]
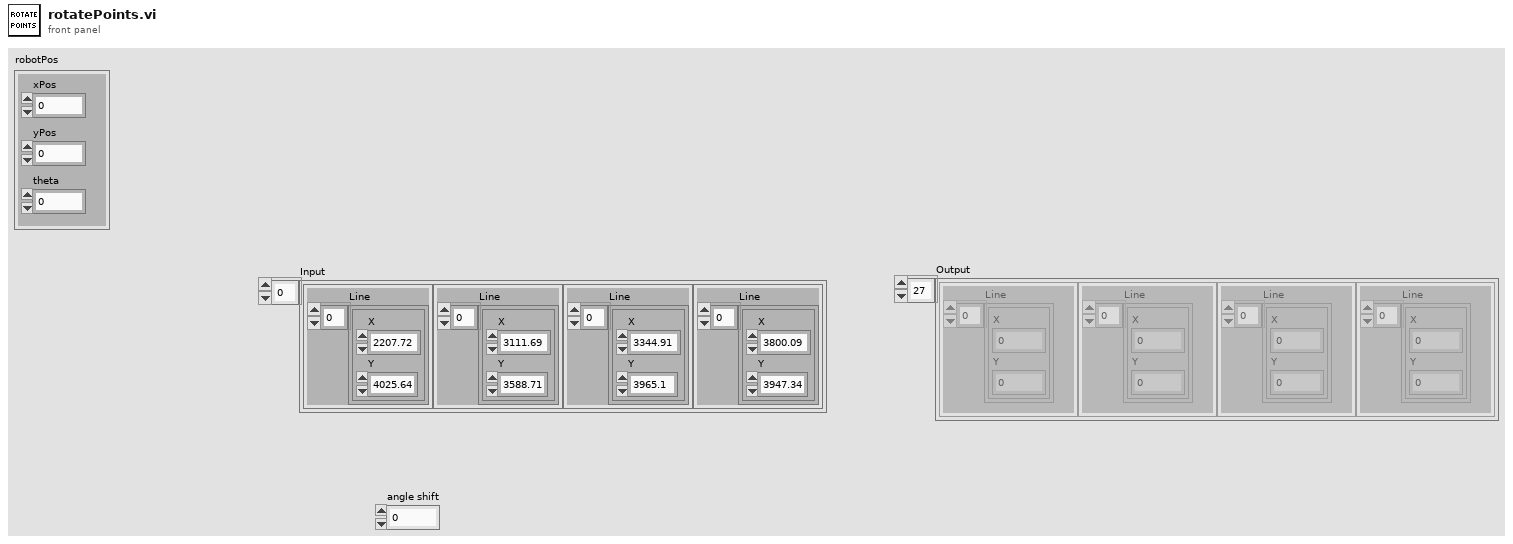
[diagram p1: front panel]
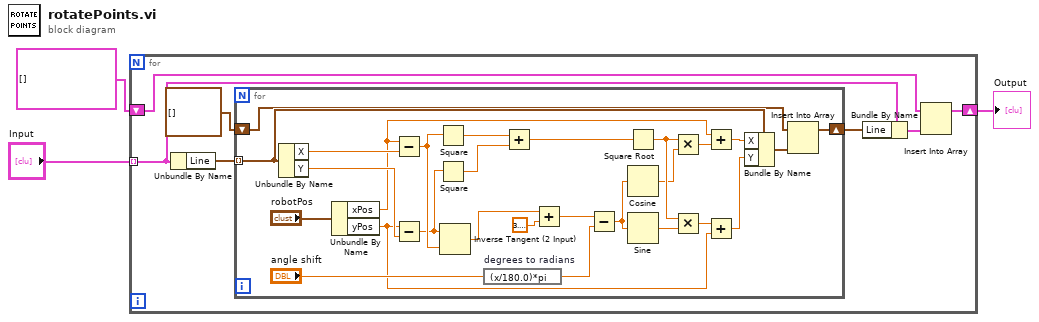
[diagram p0: block diagram]
diagram:
  n1 = for {
    tunnel: "Input" -> [w8] mode=indexing
    shift-right: [w5] -> w1
    shift-left: cluster{"Line":cluster{"X":dbl, "Y":dbl}[]}[] [] -> [w7]
    n2 = Unbundle By Name(w8) -> ("Line"=w10:cluster{"X":dbl, "Y":dbl}[])
    n3 = for {
      tunnel: w10 -> [w31] mode=indexing
      shift-right: [w30] -> w9
      shift-left: cluster{"X":dbl, "Y":dbl}[] [] -> [w28]
      n4 = Unbundle By Name(w31) -> ("X"=w20:dbl, "Y"=w19:dbl)
      n5 = Unbundle By Name("robotPos") -> ("xPos"=w16:dbl, "yPos"=w17:dbl)
      n6 = Subtract(x=w16, y=w20) -> (x-y=w24:dbl)
      n7 = Subtract(x=w17, y=w19) -> (x-y=w23:dbl)
      n8 = Square(x=w24) -> (x^2=w36:dbl)
      n9 = Square(x=w23) -> (x^2=w37:dbl)
      n10 = Inverse Tangent (2 Input)(1:w24, 2:w23) -> (0:w13:dbl)
      n11 = expression code="(x/180.0)*pi" "degrees to radians"("angle shift") -> (w15:dbl)
      n12 = Add(x=w36, y=w37) -> (x+y=w35:dbl)
      n13 = Add(x=w13, y=3.141592653589793) -> (x+y=w12:dbl)
      n14 = Subtract(x=w12, y=w15) -> (x-y=w14:dbl)
      n15 = Square Root(x=w35) -> (sqrt(x)=w33:dbl)
      n16 = Cosine(x=w14) -> (cos(x)=w25:dbl)
      n17 = Sine(x=w14) -> (sin(x)=w32:dbl)
      n18 = Multiply(x=w33, y=w25) -> (x*y=w18:dbl)
      n19 = Multiply(x=w33, y=w32) -> (x*y=w26:dbl)
      n20 = Add(x=w16, y=w18) -> (x+y=w22:dbl)
      n21 = Add(x=w26, y=w17) -> (x+y=w21:dbl)
      n22 = Bundle By Name(cluster=w31, "X"=w22, "Y"=w21) -> (w29:cluster{"X":dbl, "Y":dbl})
      n23 = Insert Into Array(array=w28, new element=w29) -> (w30:cluster{"X":dbl, "Y":dbl}[])  [unwired: 1 in]
    }
    n24 = Bundle By Name(cluster=w8, "Line"=w9) -> (w6:cluster{"Line":cluster{"X":dbl, "Y":dbl}[]})
    n25 = Insert Into Array(array=w7, new element=w6) -> (w5:cluster{"Line":cluster{"X":dbl, "Y":dbl}[]}[])  [unwired: 1 in]
  }
  "Output" <- w1
